vi "Draw_Sprite.vi"(4 "y_index":i16, 5 "SpriteBuffer":refnum<k21>="SpriteBuffer", 6 "x_index":i16, 7 "SpritesData":T1[](array[typedef])=[{"Pos_X"=0, "Pos_Y"=0, "Width"=0, "Height"=0, "BufferIndex"=0, "TransparencyColor"=0.0}, {"Pos_X"=0, "Pos_Y"=0, "Width"=0, "Height"=0, "BufferIndex"=0, "TransparencyColor"=0.0}, {"Pos_X"=0, "Pos_Y"=0, "Width"=0, "Height"=0, "BufferIndex"=0, "TransparencyColor"=0.0}], 11 "color_in":fxp<+,3,3>) -> (3 "color_out":fxp<+,3,3>)   [LabVIEW 2019, in "Sprite.lvlib"]
uses:
  Sprite.lvlib
  SpriteData.ctl
  <vilib>/rvi/DataTransferAndStorage/Container/Common/niFpgaContainerExecOnDevCompGetState.vi
  <vilib>/rvi/Emulation/niFpgaEmulationIsFPGAContextNoSignature.vi
  <vilib>/rvi/DataTransferAndStorage/Container/Common/niFpgaContainerGetUniqueNameForEmu.vi
  <vilib>/rvi/Emulation/niFpgaProcessEmulError.vi
  <vilib>/rvi/Emulation/niFpgaSctlEmulationGetInTimedLoop.vi
  <vilib>/rvi/errors/nirviReportUnexpectedCaseInternalError (U32).vi
  <vilib>/rvi/Memory/Memory_Emulation/niFpgaMemoryEmulationCacheClearOnFirstRun.vi
  <vilib>/rvi/Memory/Memory_Emulation/nirvimemoryEmulationManagerCache_MakeExclusive.vi
  <vilib>/rvi/Memory/Memory_Emulation/niFpgaMemoryEmulationValidateCache.vi
  <vilib>/rvi/Memory/Memory_Emulation/nirvimemoryEmulationManagerCache_InsertValue.vi
  <vilib>/Utility/error.llb/Clear Errors.vi
  <vilib>/rvi/Memory/Memory_Emulation/nirvimemoryEmulationManagerCache_ReleaseExclusive.vi
  <vilib>/rvi/Memory/Memory_Emulation/nirvimemoryEmulationManagerCache_GetValue.vi
  <vilib>/rvi/Memory/Memory_Emulation/nirvimemoryEmulationManagerCache_SetValue.vi
  <vilib>/rvi/Emulation/niFpgaSctlEmulationResourceMgr.vi
  <vilib>/rvi/DataTransferAndStorage/Container/XNode/niFpgaContainer.xnode
  <vilib>/rvi/Memory/Memory_Emulation/niFpgaMemoryEmulationRefIn.vi
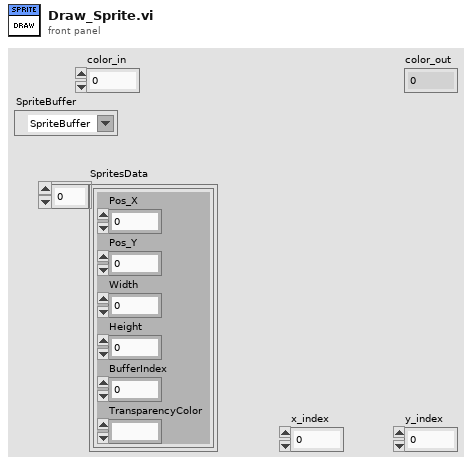
[diagram p1: front panel]
types:
  T1 = typedef "Sprite.lvlib/SpriteData.ctl" = cluster{"Pos_X":i16, "Pos_Y":i16, "Width":i16, "Height":i16, "BufferIndex":i16, "TransparencyColor":fxp<+,3,3>}
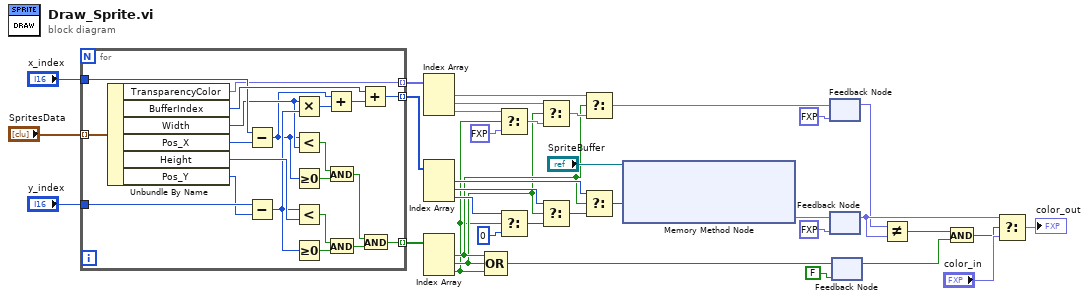
[diagram p0: block diagram]
diagram:
  n1 = for {
    tunnel: "SpritesData" -> [w57] mode=indexing
    tunnel: [w56] -> w23 mode=indexing
    tunnel: "x_index" -> [w54]
    tunnel: "y_index" -> [w52]
    tunnel: [w38] -> w22 mode=indexing
    tunnel: [w37] -> w14 mode=indexing
    n2 = Unbundle By Name(w57) -> ("TransparencyColor"=w37:fxp<+,3,3>, "BufferIndex"=w55:i16, "Width"=w41:i16, "Pos_X"=w53:i16, "Height"=w46:i16, "Pos_Y"=w51:i16)
    n3 = Subtract(x=w54, y=w53) -> (x-y=w40:i16)
    n4 = Subtract(x=w52, y=w51) -> (x-y=w42:i16)
    n5 = Multiply(x=w41, y=w42) -> (x*y=w43:i16)
    n6 = Less?(x=w40, y=w41) -> (x < y?=w49:bool)
    n7 = Greater Or Equal To 0?(x=w40) -> (x >= 0?=w50:bool)
    n8 = Less?(x=w42, y=w46) -> (x < y?=w48:bool)
    n9 = Greater Or Equal To 0?(x=w42) -> (x >= 0?=w47:bool)
    n10 = Add(x=w40, y=w43) -> (x+y=w39:i16)
    n11 = And(x=w49, y=w50) -> (x .and. y?=w45:bool)
    n12 = And(x=w48, y=w47) -> (x .and. y?=w44:bool)
    n13 = Add(x=w55, y=w39) -> (x+y=w56:i16)
    n14 = And(x=w45, y=w44) -> (x .and. y?=w38:bool)
  }
  n15 = Index Array(array=w14) -> (element #1=w6:fxp<+,3,3>, element #2=w13:fxp<+,3,3>, element #3=w7:fxp<+,3,3>)  [unwired: 3 in]
  n16 = Index Array(array=w23) -> (element #1=w4:i16, element #2=w21:i16, element #3=w5:i16)  [unwired: 3 in]
  n17 = Index Array(array=w22) -> (element #1=w3:bool, element #2=w2:bool, element #3=w1:bool)  [unwired: 3 in]
  n18 = Compound Arithmetic op=OR(w3, w2, w1) -> (w17:bool)
  n19 = Select(t=w7, s=w1, f=fxp<+,3,3> 0.0) -> (s? t:f=w15:fxp<+,3,3>)
  n20 = Select(t=w5, s=w1, f=u16 0) -> (s? t:f=w20:u16)
  n21 = Select(t=w13, s=w2, f=w15) -> (s? t:f=w16:fxp<+,3,3>)
  n22 = Select(t=w21, s=w2, f=w20) -> (s? t:f=w19:u16)
  n23 = Select(t=w6, s=w3, f=w16) -> (s? t:f=w11:fxp<+,3,3>)
  n24 = Select(t=w4, s=w3, f=w19) -> (s? t:f=w8:u16)
  n25 = xnode ("Memory Method Node")("Address"=w8, "Memory In"="SpriteBuffer") -> ("Data"=w33:fxp<+,3,3>)  [unwired: 1 out]
  n26 = feedback-in #1(w11) -> ()
  n27 = feedback #1(fxp<+,3,3> 0.0 ("f")) -> (w10:fxp<+,3,3>)
  n28 = feedback #2(fxp<+,3,3> 0.0 ("Data")) -> (w26:fxp<+,3,3>)
  n29 = feedback-in #2(w33) -> ()
  n30 = feedback-in #3(w17) -> ()
  n31 = feedback #3(FALSE) -> (w29:bool)
  n32 = Not Equal?(x=w10, y=w26) -> (x != y?=w24:bool)
  n33 = And(x=w24, y=w29) -> (x .and. y?=w25:bool)
  n34 = Select(t=w26, s=w25, f="color_in") -> (s? t:f=→"color_out":fxp<+,3,3>)
